vi "actuate_voltagePulseExp_v0.05.vi"(0 "Phase Cluster":T4, 1 "valve Time Cluster":T3, 2 "Didn't Lift?":bool, 3 "data in":T5={"daq_ao 1"="Dev1/ao0", "daq_ai 1"="Dev1/ai0", "experiment day folder"=path "D:/DATA/8-27-15 save func testing/test.lvm", "Multiclamp init error"=0, "Multiclamp Handle Out"=0, "sampling rate (Hz)"=10000, "trial name"=""}, 5 "PhaseLetter":string, 7 "controls array in":refnum<vi>[](array[refnum]), 9 "time to wait for solution change (min)":dbl=2.5 min=0.0 step=0.01, 11 "error in":errorcluster, 12 "common cluster":T7, 13 "individual controls in":T6) -> (4 "output cluster":T1, 6 "protocol waveform":waveform(dbl)[](graph), 8 "jumptestMonitor":waveform(dbl)[](graph) caption="protocol response", 10 "control array out":refnum<vi>[](array[refnum]), 14 "experiment VI ref":refnum<vi>, 15 "error out":errorcluster)   [LabVIEW 2019]
uses:
  pipette cleaning/pressure box/cleaning_soft/controls/actuator_type.ctl
  pipette cleaning/pressure box/cleaning_soft/controls/actuator_cluster.ctl
  machine_vision/coordinate model vis/transform_properties_actuators.ctl
  machine_vision/controls/transform_cluster_actuator.ctl
  controls/NH_method.ctl
  pipette cleaning/pressure box/cleaning_soft/controls/pressure_box_type.ctl
  pipette cleaning/pressure box/cleaning_soft/controls/pressure_box_control.ctl
  multipatch/controls/multipatch_common_controls_v4.ctl
  controls/memtest_def.ctl
  multipatch/controls/multipatch_individual_controls_v5.ctl
  Controls/Data.ctl
panel:
  in  "VoltageRampValuesCluster":T2
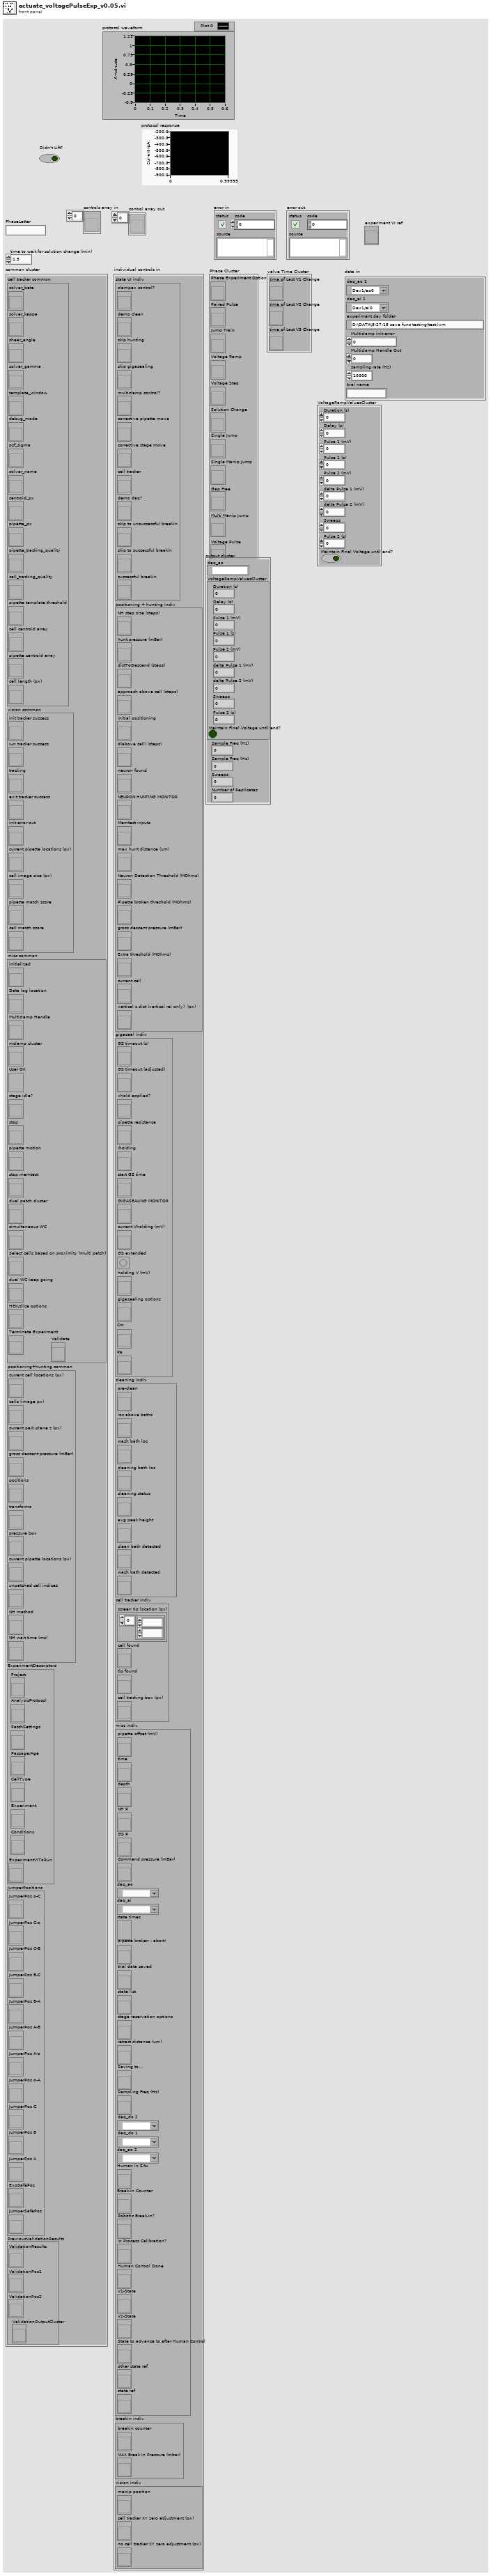
[diagram p1: front panel]
types:
  T1 = cluster{"daq_ao":tag, "VoltageRampValuesCluster":cluster{"Duration (s)":dbl, "Delay (s)":dbl, "Pulse 1 (mV)":dbl, "Pulse 1 (s)":dbl, "Pulse 2 (mV)":dbl, "delta Pulse 1 (mV)":dbl, "delta Pulse 2 (mV)":dbl, "Sweeps":dbl, "Pulse 2 (s)":dbl, "Maintain Final Voltage until end?":bool}, "Sample Freq (Hz)":dbl, "Sample Freq (Hz)":dbl, "Sweeps":dbl, "Number of Replicates":i16}
  T2 = cluster{"Duration (s)":dbl, "Delay (s)":dbl, "Pulse 1 (mV)":dbl, "Pulse 1 (s)":dbl, "Pulse 2 (mV)":dbl, "delta Pulse 1 (mV)":dbl, "delta Pulse 2 (mV)":dbl, "Sweeps":dbl, "Pulse 2 (s)":dbl, "Maintain Final Voltage until end?":bool}
  T3 = cluster{"time of Last V1 Change":refnum<vi>, "time of Last V2 Change":refnum<vi>, "time of Last V3 Change":refnum<vi>}
  T4 = cluster{"Phase Experiment Option":refnum<vi>, "Paired Pulse":refnum<vi>, "Jump Train":refnum<vi>, "Voltage Ramp":refnum<vi>, "Voltage Step":refnum<vi>, "Solution Change":refnum<vi>, "Single Jump":refnum<vi>, "Single Manip Jump":refnum<vi>, "Gap Free":refnum<vi>, "Multi Manip Jump":refnum<vi>, "Voltage Pulse":refnum<vi>, "Current Pulse":refnum<vi>, "Current Ramp":refnum<vi>, "Gap Free Iclamp":refnum<vi>}
  T5 = typedef "Data.ctl" = cluster{"daq_ao 1":tag, "daq_ai 1":tag, "experiment day folder":path, "Multiclamp init error":i32, "Multiclamp Handle Out":u32, "sampling rate (Hz)":i32, "trial name":string}
  T6 = typedef "multipatch_individual_controls_v5.ctl" = cluster{"state UI indiv":cluster{"clampex control?":refnum<vi>, "demo clean":refnum<vi>, "skip hunting":refnum<vi>, "skip gigasealing":refnum<vi>, "multiclamp control?":refnum<vi>, "corrective pipette move":refnum<vi>, "corrective stage move":refnum<vi>, "cell tracker":refnum<vi>, "demo daq?":refnum<vi>, "skip to unsuccessful breakin":refnum<vi>, "skip to successful breakin":refnum<vi>, "successful breakin":refnum<vi>}, "positioning + hunting indiv":cluster{"NH step size (steps)":refnum<vi>, "hunt pressure (mBar)":refnum<vi>, "distToDescend (steps)":refnum<vi>, "approach above cell (steps)":refnum<vi>, "initial positioning":refnum<vi>, "d(above cell) (steps)":refnum<vi>, "neuron found":refnum<vi>, "NEURON HUNTING MONITOR":refnum<vi>, "Memtest inputs":refnum<vi>, "max hunt distance (um)":refnum<vi>, "Neuron Detection Threshold (MOhms)":refnum<vi>, "Pipette broken threshold (MOhms)":refnum<vi>, "gross descent pressure (mBar)":refnum<vi>, "Extra threshold (MOhms)":refnum<vi>, "current cell":refnum<vi>, "vertical z dist (vertical rel only)  (px)":refnum<vi>}, "gigaseal indiv":cluster{"GS timeout (s)":refnum<vi>, "GS timeout (adjusted)":refnum<vi>, "vhold applied?":refnum<vi>, "pipette resistance":refnum<vi>, "Iholding":refnum<vi>, "start GS time":refnum<vi>, "GIGASEALING MONITOR":refnum<vi>, "current Vholding (mV)":refnum<vi>, "GS extended":refnum<vi>, "holding V (mV)":refnum<vi>, "gigasealing options":refnum<vi>, "Cm":refnum<vi>, "Ra ":refnum<vi>}, "cleaning indiv":cluster{"pre-clean":refnum<vi>, "loc above baths":refnum<vi>, "wash bath loc":refnum<vi>, "cleaning bath loc":refnum<vi>, "cleaning status":refnum<vi>, "avg peak height":refnum<vi>, "clean bath detected":refnum<vi>, "wash bath detected":refnum<vi>}, "cell tracker indiv":cluster{"screen tip location (px)":refnum<vi>, "cell found":refnum<vi>, "tip found":refnum<vi>, "cell tracking box (px)":refnum<vi>}, "misc indiv":cluster{"pipette offset (mV)":refnum<vi>, "time":refnum<vi>, "depth":refnum<vi>, "NH R":refnum<vi>, "GS R":refnum<vi>, "Command pressure (mBar)":refnum<vi>, "daq_ao":tag, "daq_ai":tag, "state times":refnum<vi>, "pipette broken - abort!":refnum<vi>, "trial data saved":refnum<vi>, "state list":refnum<vi>, "stage reservation options":refnum<vi>, "retract distance (um)":refnum<vi>, "Saving to...":refnum<vi>, "Sampling Freq (Hz)":refnum<vi>, "daq_do 2":tag, "daq_do 1":tag, "daq_ao 2":tag, "Human in Situ":refnum<vi>, "Break-In Counter":refnum<vi>, "Robotic Break-In?":refnum<vi>, "In Process Calibration?":refnum<vi>, "Human Control Done":refnum<vi>, "V1-State":refnum<vi>, "V2-State":refnum<vi>, "State to advance to after Human Control":refnum<vi>, "other state ref":refnum<vi>, "state ref":refnum<vi>}, "breakin indiv":cluster{"breakin counter":refnum<vi>, "MAX Break In Pressure (mbar)":refnum<vi>}, "vision indiv":cluster{"manip position":refnum<vi>, "cell tracker XY zero adjustment (px)":refnum<vi>, "no cell tracker XY zero adjustment (px)":refnum<vi>}}
  T7 = typedef "multipatch_common_controls_v4.ctl" = cluster{"cell tracker common":cluster{"solver_beta":refnum<vi>, "solver_kappa":refnum<vi>, "shear_angle":refnum<vi>, "solver_gamma":refnum<vi>, "template_window":refnum<vi>, "debug_mode":refnum<vi>, "psf_sigma":refnum<vi>, "solver_name":refnum<vi>, "centroid_px":refnum<vi>, "pipette_px":refnum<vi>, "pipette_tracking_quality":refnum<vi>, "cell_tracking_quality":refnum<vi>, "pipette template threshold":refnum<vi>, "cell centroid array":refnum<vi>, "pipette centroid array":refnum<vi>, "cell length (px)":refnum<vi>}, "vision common":cluster{"init tracker success":refnum<vi>, "run tracker success":refnum<vi>, "tracking":refnum<vi>, "exit tracker success":refnum<vi>, "init error out":refnum<vi>, "current pipette locations (px)":refnum<vi>, "cell image size (px)":refnum<vi>, "pipette match score":refnum<vi>, "cell match score":refnum<vi>}, "misc common":cluster{"initialized":refnum<vi>, "Data log location":refnum<vi>, "Multiclamp Handle":refnum<vi>, "mclamp cluster":refnum<vi>, "User OK":refnum<vi>, "stage idle?":refnum<vi>, "stop":refnum<vi>, "pipette motion":refnum<vi>, "stop memtest":refnum<vi>, "dual patch cluster":refnum<vi>, "simultaneous WC":refnum<vi>, "Select cells based on proximity (multi patch)":refnum<vi>, "dual WC keep going":refnum<vi>, "HEK/slice options":refnum<vi>, "Terminate Experiment":refnum<vi>, "Validate":refnum<vi>}, "positioning+hunting common":cluster{"current cell locations (px)":refnum<vi>, "cells (image px)":refnum<vi>, "current park plane z (px)":refnum<vi>, "gross descent pressure (mBar)":refnum<vi>, "positions":refnum<vi>, "transforms":refnum<vi>, "pressure box":refnum<vi>, "current pipette locations (px)":refnum<vi>, "unpatched cell indices":refnum<vi>, "NH method":refnum<vi>, "NH wait time (ms)":refnum<vi>}, "ExperimentDescriptors":cluster{"Project":refnum<vi>, "AnalysisProtocol":refnum<vi>, "PatchSettings":refnum<vi>, "Passage/Age":refnum<vi>, "CellType":refnum<vi>, "Experiment":refnum<vi>, "Conditions":refnum<vi>, "ExperimentVIToRun":refnum<vi>}, "JumperPositions":cluster{"JumperPos o-C":refnum<vi>, "JumperPos C-o":refnum<vi>, "JumperPos C-B":refnum<vi>, "JumperPos B-C":refnum<vi>, "JumperPos B-A":refnum<vi>, "JumperPos A-B":refnum<vi>, "JumperPos A-o":refnum<vi>, "JumperPos o-A":refnum<vi>, "JumperPos C":refnum<vi>, "JumperPos B":refnum<vi>, "JumperPos A":refnum<vi>, "ExpSafePos":refnum<vi>, "jumperSafePos":refnum<vi>}, "PreviousValidationResults":cluster{"ValidationResults":refnum<vi>, "ValidationPos1":refnum<vi>, "ValidationPos2":refnum<vi>, "ValidationOutputCluster":refnum<vi>}}
  T8 = cluster{"Which Position to use for Experiment":enum16{"Jumper Safe Position", "Experiment Safe Position", "Jumper Position A", "Jumper Position B", "Jumper Position C", "Jumper Position o-A", "Jumper Position A-o", "Jumper Position A-B", "Jumper Position B-A", "Jumper Position B-C", "Jumper Position C-B", "Jumper Position C-o", "Jumper Position o-C", "Don't Move"}, "Duration (s)":dbl, "Delay (s)":dbl, "Pulse 2 (s)":dbl, "Pulse 1 (mV)":dbl, "Replicates":dbl, "Pulse 1 (s)":dbl, "Pulse 2 (mV)":dbl, "Vholding (mV)":dbl, "Valve 1 Position":i16, "Valve 2 Position":i16, "Valve 3 Position":i16, "valve 1 used now?":bool, "valve 2 used now?":bool, "valve 3 used now? ":bool, "Maintain Final Voltage until end?":bool, "delta Pulse 1 (mV)":dbl, "delta Pulse 2 (mV)":dbl, "Sweeps":dbl, "Final Pulse 1 (mV)":dbl, "Final Pulse 2 (mV)":dbl, "protocol Preview":waveform(dbl)[]}
  T9 = enum16{"Jumper Safe Position", "Experiment Safe Position", "Jumper Position A", "Jumper Position B", "Jumper Position C", "Jumper Position o-A", "Jumper Position A-o", "Jumper Position A-B", "Jumper Position B-A", "Jumper Position B-C", "Jumper Position C-B", "Jumper Position C-o", "Jumper Position o-C", "Don't Move"}
  T10 = enum16{"manipulator 1", "manipulator 2", "manipulator 3", "manipulator 4"}
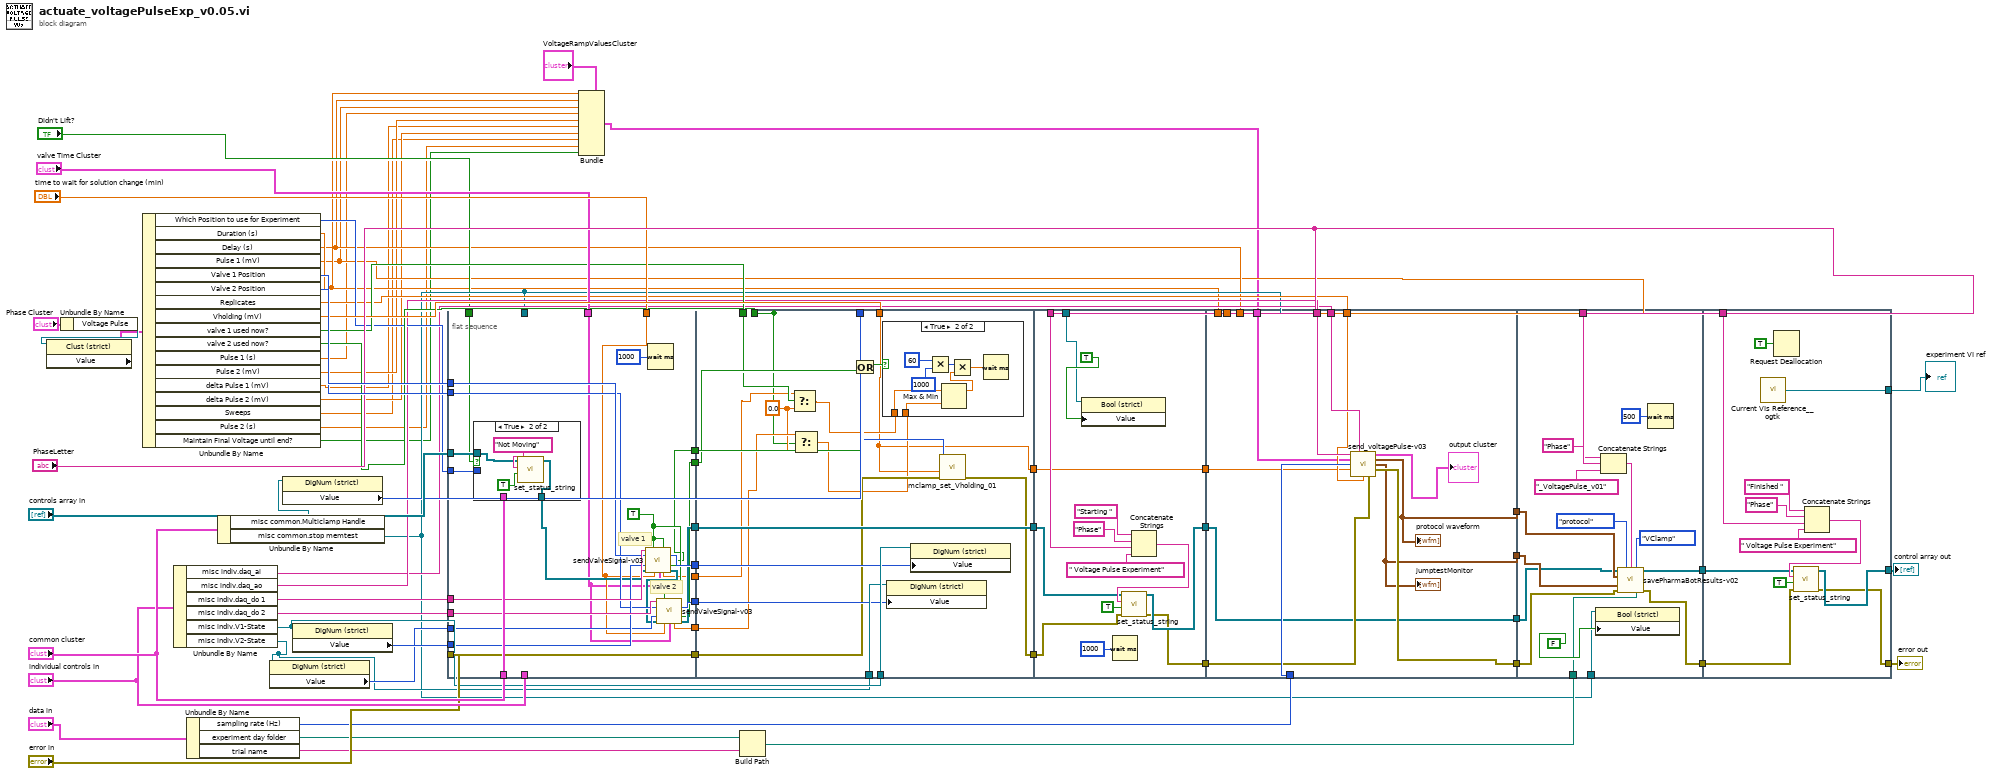
[diagram p0: block diagram]
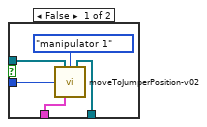
[diagram p2: hidden frame]
diagram:
  n1 = Unbundle By Name("Phase Cluster") -> ("Voltage Pulse"=w47:refnum<vi>)
  n2 = property class="Clust (strict)"(reference=w47) -> ("Value"=w46:T8)  [unwired: 1 in, 2 out]
  n3 = Unbundle By Name(w46) -> ("Which Position to use for Experiment"=w22:T9, "Duration (s)"=w15:dbl, "Delay (s)"=w14:dbl, "Pulse 1 (mV)"=w13:dbl, "Valve 1 Position"=w45:i16, "Valve 2 Position"=w44:i16, "Replicates"=w21:dbl, "Vholding (mV)"=w31:dbl, "valve 1 used now?"=w24:bool, "valve 2 used now?"=w23:bool, "Pulse 1 (s)"=w12:dbl, "Pulse 2 (mV)"=w11:dbl, "delta Pulse 1 (mV)"=w7:dbl, "delta Pulse 2 (mV)"=w6:dbl, "Sweeps"=w5:dbl, "Pulse 2 (s)"=w4:dbl, "Maintain Final Voltage until end?"=w3:bool)
  n4 = Unbundle By Name("individual controls in") -> ("misc indiv.daq_ai"=w18:tag, "misc indiv.daq_ao"=w19:tag, "misc indiv.daq_do 1"=w67:tag, "misc indiv.daq_do 2"=w66:tag, "misc indiv.V1-State"=w58:refnum<vi>, "misc indiv.V2-State"=w57:refnum<vi>)
  n5 = Unbundle By Name("data in") -> ("sampling rate (Hz)"=w20:i32, "experiment day folder"=w51:path, "trial name"=w50:string)
  n6 = Unbundle By Name("common cluster") -> ("misc common.Multiclamp Handle"=w30:refnum<vi>, "misc common.stop memtest"=w17:refnum<vi>)
  n7 = property class="DigNum (strict)"(reference=w57) -> ("Value"=w59:u16)  [unwired: 1 in, 2 out]
  n8 = property class="DigNum (strict)"(reference=w30) -> ("Value"=w29:u32)  [unwired: 1 in, 2 out]
  n9 = property class="DigNum (strict)"(reference=w58) -> ("Value"=w60:u16)  [unwired: 1 in, 2 out]
  n10 = flat-sequence {
    tunnel: "common cluster" -> [w92]
    tunnel: "individual controls in" -> [_]
    tunnel: [w89] -> w62
    tunnel: [w86] -> w56
    tunnel: [w85] -> w55
    tunnel: [w79] -> w38
    tunnel: [w77] -> w33
    tunnel: [w76] -> w32
    tunnel: "time to wait for solution change (min)" -> [w75]
    tunnel: "valve Time Cluster" -> [w74]
    tunnel: [w73] -> w26
    tunnel: [w72] -> w25
    tunnel: w17 -> [_]
    tunnel: "Didn't Lift?" -> [w70]
    tunnel: w22 -> [w93]
    tunnel: w67 -> [w91]
    tunnel: w66 -> [w90]
    tunnel: "error in" -> [w89]
    tunnel: w60 -> [w88]
    tunnel: w59 -> [w87]
    tunnel: w45 -> [w84]
    tunnel: w44 -> [w83]
    tunnel: "controls array in" -> [w82]
    tunnel: [w111] -> w63
    tunnel: w62 -> [w113]
    tunnel: w58 -> [w121]
    tunnel: w57 -> [w120]
    tunnel: w56 -> [w119]
    tunnel: w55 -> [w118]
    tunnel: [w117] -> w39
    tunnel: w38 -> [w117]
    tunnel: w33 -> [w115]
    tunnel: w32 -> [w114]
    tunnel: w31 -> [w103]
    tunnel: w29 -> [w112]
    tunnel: w26 -> [w108]
    tunnel: w25 -> [w107]
    tunnel: w24 -> [w109]
    tunnel: [w104] -> _
    tunnel: w23 -> [w104]
    tunnel: [w103] -> w8
    tunnel: w17 -> [w130]
    tunnel: [w132] -> w64
    tunnel: w63 -> [w133]
    tunnel: [w134] -> w40
    tunnel: w39 -> [w135]
    tunnel: "PhaseLetter" -> [w136]
    tunnel: [w129] -> w9
    tunnel: w8 -> [w129]
    tunnel: w18 -> [w154]
    tunnel: w19 -> [w153]
    tunnel: w64 -> [w148]
    tunnel: [w151] -> w54
    tunnel: [w145] -> w53
    tunnel: w21 -> [w149]
    tunnel: w15 -> [_]
    tunnel: w20 -> [w150]
    tunnel: w13 -> [_]
    tunnel: w14 -> [_]
    tunnel: [w147] -> w43
    tunnel: [w146] -> w41
    tunnel: w40 -> [w146]
    tunnel: w10 -> [w143]
    tunnel: w9 -> [w144]
    tunnel: w17 -> [w169]
    tunnel: w54 -> [w168]
    tunnel: w53 -> [w167]
    tunnel: w49 -> [w164]
    tunnel: "PhaseLetter" -> [w162]
    tunnel: w43 -> [w159]
    tunnel: w41 -> [w158]
    tunnel: [w156] -> w36
    tunnel: [w157] -> w35
    tunnel: [w176] -> w37
    tunnel: [w175] -> w61
    tunnel: w36 -> [w174]
    tunnel: w35 -> [w177]
    tunnel: "PhaseLetter" -> [w173]
    tunnel: [w172] -> w1
    frame #0 {
      w78 = TRUE ("Set Status")
      # "valve 2"
      # "valve 1"
      n11 = case shown="True" w70 {
        tunnel: w93 -> [w98 _]
        tunnel: w92 -> [w97 _]
        tunnel: w82 -> [w95 w99]
        tunnel: [w94 w100] -> w81
        frame False {
          n12 = call "moveToJumperPosition-v02.vi"("which manipulator"=T10."manipulator 1", "controls array in"=w95, "Which Jumper Position to move to?"=w98, "common cluster"=w97) -> ("control array out"=w94:refnum<vi>[])  [unwired: 10 in, 1 out]
        }
        frame True {
          n13 = call "set_status_string.vi"("new line?"=TRUE, "status string in"="Not Moving", "controls array"=w99) -> ("controls array out"=w100:refnum<vi>[])  [unwired: 7 in, 1 out]
        }
      }
      n14 = call "sendValveSignal-v03.vi"("daq_do"=w91, "Set Status"=w78, "Valve1?"=w78, "ChangeToValve"=w84, "CurrentValve"=w88, "controls array in"=w81, "time to wait for solution change (min)"=w75, "valve Time Cluster"=w74) -> ("ValveSetTo"=w85:u16, "valve changed?"=w77:bool, "additional time to wait (min)"=w73:dbl, "control array out"=w80:refnum<vi>[])  [unwired: 4 in]
      n15 = Wait (ms)(milliseconds to wait=u32 1000) -> ()  [unwired: 1 out]
      n16 = call "sendValveSignal-v03.vi"("daq_do"=w90, "Set Status"=w78, "ChangeToValve"=w83, "CurrentValve"=w87, "controls array in"=w80, "time to wait for solution change (min)"=w75, "valve Time Cluster"=w74) -> ("ValveSetTo"=w86:u16, "valve changed?"=w76:bool, "additional time to wait (min)"=w72:dbl, "control array out"=w79:refnum<vi>[])  [unwired: 5 in]
    }
    frame #1 {
      w105 = 0.0 ("f")
      n17 = Select(t=w108, s=w109, f=w105) -> (s? t:f=w110:dbl)
      n18 = Select(t=w107, s=w104, f=w105) -> (s? t:f=w106:dbl)
      n19 = Or(x=w115, y=w114) -> (x .or. y?=w116:bool)
      n20 = case shown="True" w116 {
        tunnel: w110 -> [_ w124]
        tunnel: w106 -> [_ w123]
        frame False {
        }
        frame True {
          n21 = Multiply(x=u32 60 ("milliseconds to wait"), y=u32 1000) -> (x*y=w126:u32)
          n22 = Max & Min(x=w124, y=w123) -> (max(x,y)=w122:dbl)  [unwired: 1 out]
          n23 = Multiply(x=w126, y=w122) -> (x*y=w125:dbl)
          n24 = Wait (ms)(milliseconds to wait=w125) -> ()  [unwired: 1 out]
        }
      }
      n25 = property class="DigNum (strict)"(reference=w120, "Value"=w119) -> ()  [unwired: 1 in, 2 out]
      n26 = property class="DigNum (strict)"(reference=w121, "Value"=w118) -> ()  [unwired: 1 in, 2 out]
      n27 = call "mclamp_set_Vholding_01.vi"("error in (no error)"=w113, "set holding (mV)"=w103, "Multiclamp Handle Out"=w112) -> ("error out"=w111:errorcluster)  [unwired: 7 in, 1 out]
    }
    frame #2 {
      n28 = property class="Bool (strict)"(reference=w130, "Value"=TRUE ("stop memtest")) -> ()  [unwired: 1 in, 2 out]
      n29 = Wait (ms)(milliseconds to wait=u32 1000) -> ()  [unwired: 1 out]
      n30 = Concatenate Strings("Starting " ("string"), "Phase" ("string"), w136, " Voltage Pulse Experiment" ("string")) -> (w138:string)
      n31 = call "set_status_string.vi"("error in"=w133, "new line?"=TRUE, "status string in"=w138, "controls array"=w135) -> ("error out"=w132:errorcluster, "controls array out"=w134:refnum<vi>[])  [unwired: 6 in]
    }
    frame #3 {
      n32 = call "send_voltagePulse-v03.vi"("daq_ao"=w153, "daq_ai"=w154, "VoltageRampValuesCluster"=w143, "Sample Freq (Hz)"=w150, "set holding (mV)"=w144, "Number of Replicates"=w149, "error in"=w148) -> ("output cluster"=→"output cluster":T1, "output waveform"=w151:waveform(dbl)[], "protocol response"=w145:waveform(dbl)[], "error out"=w147:errorcluster)  [unwired: 5 in]
      "jumptestMonitor" <- w145
      "protocol waveform" <- w151
    }
    frame #4 {
      n33 = property class="Bool (strict)"(reference=w169, "Value"=FALSE ("stop memtest")) -> ()  [unwired: 1 in, 2 out]
      n34 = Concatenate Strings("Phase" ("string"), w162, "_VoltagePulse_v01" ("string")) -> (w163:string)
      n35 = call "savePharmaBotResults-v02.vi"("controls array"=w158, "protocol or memtest"=enum16{"protocol", "memtest", "validation"}."protocol", "ExpPhase"=w163, "which clamp"=enum16{"VClamp", "IClamp"}."VClamp", "protocol waveform"=w168, "protocol response"=w167, "error in"=w159, "Save to (folder dir)"=w164) -> ("controls array out"=w157:refnum<vi>[], "error out"=w156:errorcluster)  [unwired: 6 in]
      n36 = Wait (ms)(milliseconds to wait=u32 500) -> ()  [unwired: 1 out]
    }
    frame #5 {
      n37 = call "Current VIs Reference__ogtk.vi"() -> ("Current VI's reference"=w172:refnum<vi>)  [unwired: 5 in]
      n38 = Request Deallocation(TRUE ("flag")) -> ()
      n39 = Concatenate Strings("Finished " ("string"), "Phase" ("string"), w173, " Voltage Pulse Experiment" ("string")) -> (w179:string)
      n40 = call "set_status_string.vi"("error in"=w174, "new line?"=TRUE, "status string in"=w179, "controls array"=w177) -> ("error out"=w175:errorcluster, "controls array out"=w176:refnum<vi>[])  [unwired: 6 in]
    }
  }
  n41 = Bundle(cluster="VoltageRampValuesCluster", "Duration (s)"=w15, "Delay (s)"=w14, "Pulse 1 (mV)"=w13, "Pulse 1 (s)"=w12, "Pulse 2 (mV)"=w11, "delta Pulse 1 (mV)"=w7, "delta Pulse 2 (mV)"=w6, "Sweeps"=w5, "Pulse 2 (s)"=w4, "Maintain Final Voltage until end?"=w3) -> (w10:T2)
  n42 = Build Path(base path=w51, name or relative path=w50) -> (appended path=w49:path)
  "error out" <- w61
  "control array out" <- w37
  "experiment VI ref" <- w1
